vi "servo_oven_heater.vi"() -> ()   [LabVIEW 2015]
uses:
  <vilib>/addons/control/pid/pid.llb/PID Advanced (DBL).vi
  <vilib>/addons/control/pid/NI_PID_pid.lvlib
panel:
  in  "dt (s)":dbl=1.0 format="%.3f"
  in  "PID Gains":T1={"proportional gain (Kc)"=8.5, "integral time (Ti, min)"=2.3, "derivative time (Td, min)"=0.35} {"derivative time (Td, min)" format="%#.6g"; "integral time (Ti, min)" format="%#.6g"; "proportional gain (Kc)" format="%#.6g"}
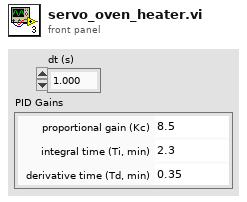
[diagram p1: front panel]
types:
  T1 = cluster{"proportional gain (Kc)":dbl, "integral time (Ti, min)":dbl, "derivative time (Td, min)":dbl}
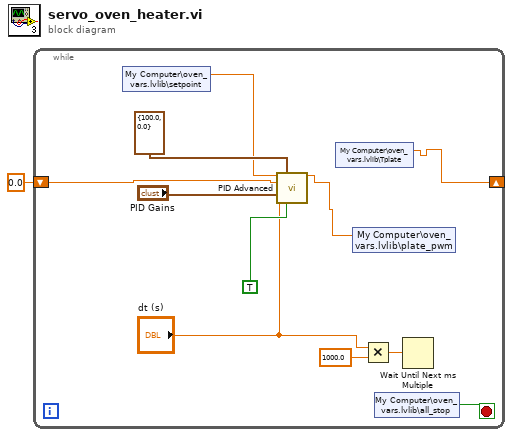
[diagram p0: block diagram]
diagram:
  n1 = while {
    shift-right: [w4] -> _
    shift-left: 0.0 ("Double") -> [w6]
    stop <- w3 stop-if-true
    n2 = shared-variable "My Computer\\oven_vars.lvlib\\setpoint"() -> (w2:dbl)  [unwired: 1 in, 1 out]
    n3 = call-poly <vilib>:"PID Advanced.vi"("setpoint"=w2, "output range"=cluster{"output high":dbl, "output low":dbl} {"output high"=100.0, "output low"=0.0}, "process variable"=w6, "PID gains"="PID Gains", "dt (s)"="dt (s)", "reinitialize? (F)"=TRUE) -> ("output"=w5:dbl)  [unwired: 8 in, 1 out]
    n4 = shared-variable "My Computer\\oven_vars.lvlib\\Tplate"() -> (w4:dbl)  [unwired: 1 in, 1 out]
    n5 = shared-variable "My Computer\\oven_vars.lvlib\\plate_pwm"(w5) -> ()  [unwired: 1 in, 1 out]
    n6 = Multiply(x="dt (s)", y=1000.0) -> (x*y=w9:dbl)
    n7 = shared-variable "My Computer\\oven_vars.lvlib\\all_stop"() -> (w3:bool)  [unwired: 1 in, 1 out]
    n8 = Wait Until Next ms Multiple(millisecond multiple=w9) -> ()  [unwired: 1 out]
  }
